vi "I will save.vi"() -> ()   [LabVIEW 2024]
panel:
  in  "Numeric":i32
  out "Numeric 2":dbl
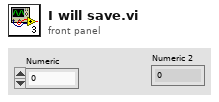
[diagram p1: front panel]
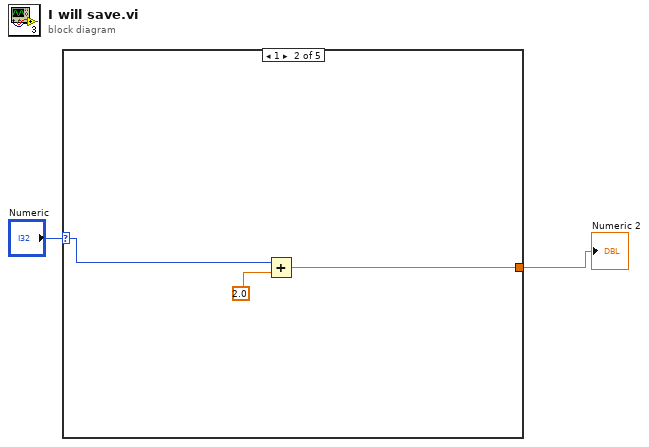
[diagram p0: block diagram]
diagram:
  n1 = case shown="1" "Numeric" {
    selector: "Numeric" -> [_ w4 _ _ _]
    tunnel: [_ w3 _ _ _] -> w2
    frame 0, Default {
    }
    frame 1 {
      n2 = Add(x=w4, y=2.0) -> (x+y=w3:dbl)
    }
    frame 5 {
    }
    frame 7 {
    }
    frame 10 {
    }
  }
  "Numeric 2" <- w2
